vi "Limelight Lock(Turret).vi"(8 "Turret Angle":dbl) -> (0 "Target Angle":dbl)   [LabVIEW 2019]
uses:
  <vilib>/Rock Robotics/Network Tables/NT Read Number.vi
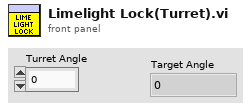
[diagram p1: front panel]
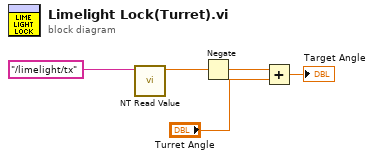
[diagram p0: block diagram]
diagram:
  n1 = call-poly <vilib>:"NT Read Value.vi"("Name"="/limelight/tx") -> ("Numeric"=w4:dbl)  [unwired: 9 in, 1 out]
  n2 = Negate(x=w4) -> (-x=w1:dbl)
  n3 = Add(x=w1, y="Turret Angle") -> (x+y=→"Target Angle":dbl)
